vi "SendToBL_WeldAuto_Recipe.vi"(0 "connection ID":refnum<k5>, 1 "SC parameter to BL":string, 2 "MessageID_SC":i32, 7 "MessageID_PC_AC":i32, 9 "ResponseID":u8=66, 11 "Error IN":errorcluster, 12 "PC_AC parameter to BL":string) -> (4 "connection ID":refnum<k5>, 6 "Test status":string=" Success", 8 "String value response":string, 10 "Error OUT":errorcluster, 14 "SC Parameter written":i32, 15 "PC_AC parameter written":i32)   [LabVIEW 2017]
panel:
  out "*(type *) &x 2":u8
  out "*(type *) &x":u8
  # "INPUT"
  # "OUTPUT"
  # "Just for reference. Hence disabled"
  # "Read Me:\nThis VI will send the set of recipe parameters to \nSC BL and verifies the response recieved from the SCBL"
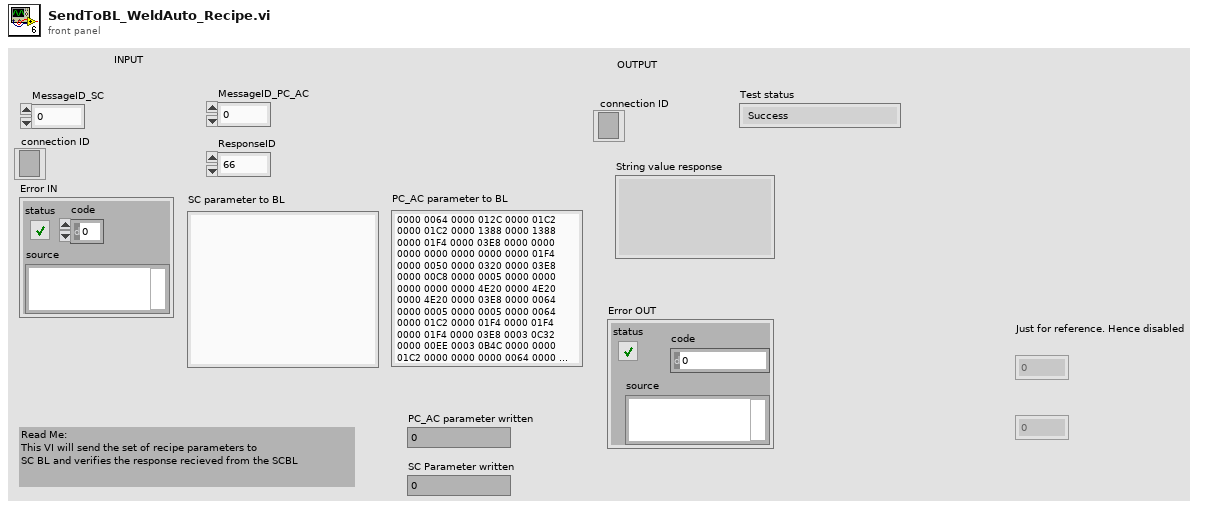
[diagram p1: front panel]
types:
  T1 = enum16{"big-endian, network order", "native, host order", "little-endian"}
  T2 = cluster{"SC parameter to BL":string, i32, "MessageID_SC":i32}
  T3 = cluster{"PC_AC parameter to BL":string, i32, "MessageID_PC_AC":i32}
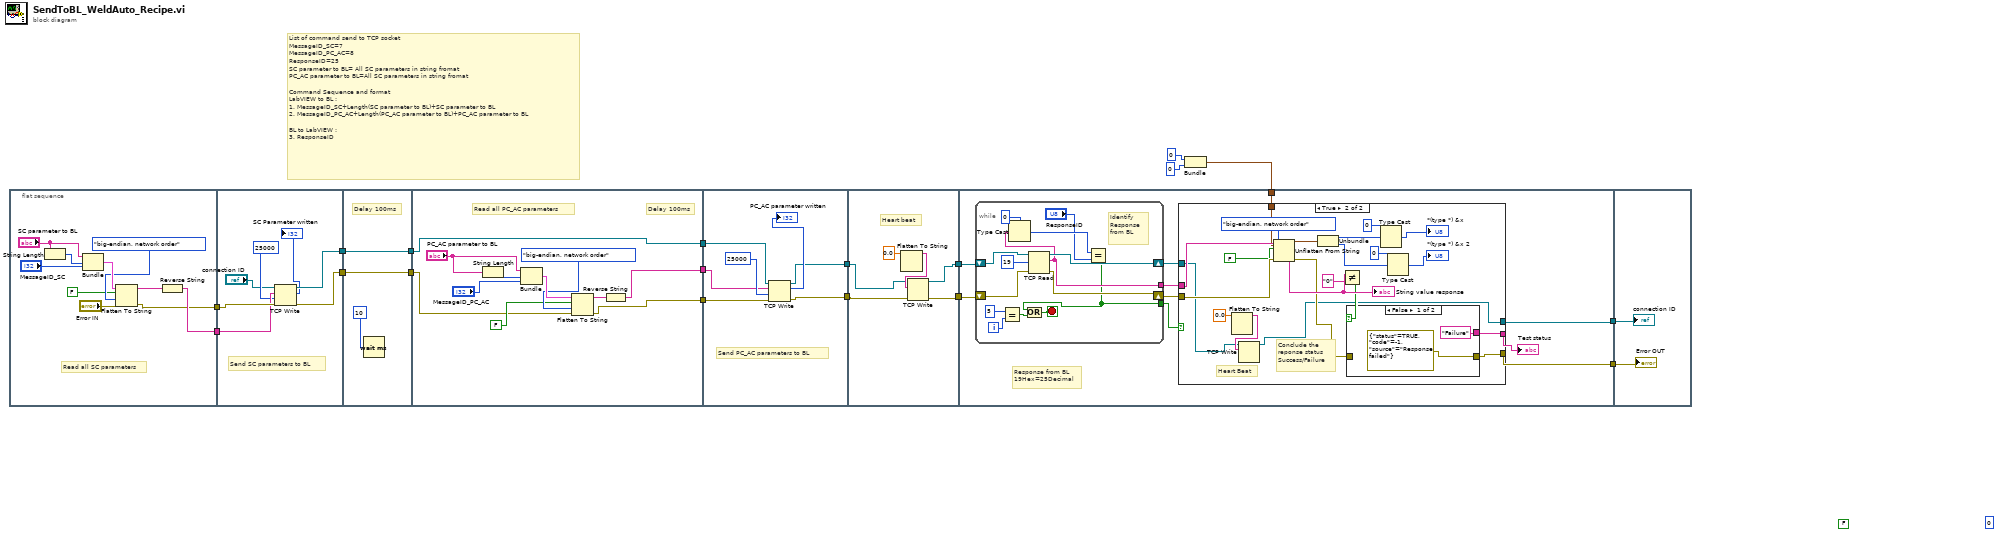
[diagram p0: block diagram]
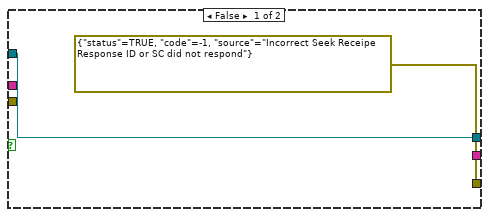
[diagram p2: hidden frame]
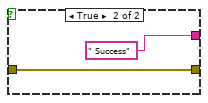
[diagram p3: hidden frame]
diagram:
  (unwired) u8 0
  (unwired) FALSE ("data includes array or string size? (T)")
  # "List of command send to TCP socket\nMessageID_SC=7\nMessageID_PC_AC=8\nResponseID=25\nSC parameter to BL= All SC parameters in string fromat\nPC_AC parameter to BL=All SC parameters in string fromat\n\nCommand Sequence and format\nLabVIEW to BL :\n1. MessageID_SC+Length(SC parameter to BL)+SC parameter to BL\n2. MessageID_PC_AC+Length(PC_AC parameter to BL)+PC_AC parameter to BL\n\nBL to LabVIEW :\n3. ResponseID"
  n1 = flat-sequence {
    tunnel: [w21] -> w11
    tunnel: [w22] -> w10
    tunnel: [w35] -> w18
    tunnel: [w34] -> w17
    tunnel: w11 -> [w33]
    tunnel: w10 -> [w32]
    tunnel: w18 -> [w38]
    tunnel: w17 -> [w37]
    tunnel: [w38] -> w9
    tunnel: [w37] -> w8
    tunnel: [w49] -> w7
    tunnel: [w48] -> w6
    tunnel: [w47] -> w5
    tunnel: w8 -> [w39]
    tunnel: w9 -> [w49]
    tunnel: [w51] -> w4
    tunnel: [w50] -> w2
    tunnel: w7 -> [w54]
    tunnel: w6 -> [w53]
    tunnel: w5 -> [w52]
    tunnel: w4 -> [w60]
    tunnel: [w58] -> w3
    tunnel: w2 -> [w59]
    tunnel: [w57] -> w1
    tunnel: w3 -> [w72]
    tunnel: w1 -> [w71]
    tunnel: w14 -> [w66]
    tunnel: [w65] -> w13
    tunnel: [w64] -> w12
    tunnel: w13 -> [w116]
    tunnel: w12 -> [w115]
    frame #0 {
      # "Read all SC parameters"
      n2 = String Length(string="SC parameter to BL") -> (length=w20:i32)
      n3 = Bundle("SC parameter to BL"="SC parameter to BL", w20, "MessageID_SC"="MessageID_SC") -> (w28:T2)  [unwired: 1 in]
      n4 = Flatten To String(anything=w28, prepend array or string size? (T)=FALSE, byte order (0:big-endian, network order)=T1."big-endian, network order", error in (no error)="Error IN") -> (data string=w25:string, error out=w21:errorcluster)  [unwired: 1 out]
      n5 = Reverse String(1:w25) -> (0:w22:string)
    }
    frame #1 {
      # "Send SC parameters to BL"
      n6 = TCP Write(connection ID="connection ID", data in=w32, error in (no error)=w33, 9:25000 ("timeout ms (25000)")) -> (connection ID out=w35:refnum<k5>, bytes written=→"SC Parameter written":i32, error out=w34:errorcluster)
    }
    frame #2 {
      # "Delay 100ms"
      n7 = Wait (ms)(milliseconds to wait=u32 10) -> ()  [unwired: 1 out]
    }
    frame #3 {
      # "Read all PC_AC parameters"
      # "Delay 100ms"
      n8 = String Length(string="PC_AC parameter to BL") -> (length=w41:i32)
      n9 = Bundle("PC_AC parameter to BL"="PC_AC parameter to BL", w41, "MessageID_PC_AC"="MessageID_PC_AC") -> (w46:T3)  [unwired: 1 in]
      n10 = Flatten To String(anything=w46, prepend array or string size? (T)=FALSE, byte order (0:big-endian, network order)=T1."big-endian, network order", error in (no error)=w39) -> (data string=w44:string, error out=w48:errorcluster)  [unwired: 1 out]
      n11 = Reverse String(1:w44) -> (0:w47:string)
    }
    frame #4 {
      # "Send PC_AC parameters to BL"
      n12 = TCP Write(connection ID=w54, data in=w52, error in (no error)=w53, 9:25000 ("timeout ms (25000)")) -> (connection ID out=w51:refnum<k5>, bytes written=→"PC_AC parameter written":i32, error out=w50:errorcluster)
    }
    frame #5 {
      # "Heart beat"
      n13 = Flatten To String(anything=0.0) -> (data string=w61:string)  [unwired: 3 in, 2 out]
      n14 = TCP Write(connection ID=w60, data in=w61, error in (no error)=w59) -> (connection ID out=w58:refnum<k5>, error out=w57:errorcluster)  [unwired: 1 in, 1 out]
    }
    frame #6 {
      # "Response from BL\n19Hex=25Decimal"
      n15 = while {
        tunnel: [w110] -> w69
        shift-right: [w112] -> w68
        shift-left: w72 -> [w114]
        shift-right: [w106] -> w70
        shift-left: w71 -> [w113]
        tunnel: [w104] -> w67
        i -> [w103]
        stop <- w105 stop-if-true
        # "Identify\nResponse \nfrom BL"
        n16 = Equal?(x=5, y=w103) -> (x = y?=w101:bool)
        n17 = TCP Read(connection ID=w114, bytes to read=19, error in (no error)=w113) -> (connection ID out=w112:refnum<k5>, data out=w110:string, error out=w106:errorcluster)  [unwired: 2 in]
        n18 = Type Cast(type=u8 0, x=w110) -> (*(type *) &x=w108:u8)
        n19 = Equal?(x=w108, y="ResponseID") -> (x = y?=w104:bool)
        n20 = Or(x=w104, y=w101) -> (x .or. y?=w105:bool)
      }
      n21 = case shown="True" w67 {
        tunnel: w70 -> [_ w96]
        tunnel: w69 -> [_ w95]
        tunnel: w68 -> [w74 w76]
        tunnel: w66 -> [_ w91]
        tunnel: [w74 w75] -> w65
        tunnel: [errorcluster {"status"=TRUE, "code"=-1, "source"="Incorrect Seek Receipe Response ID or SC did not respond"} ("error constant") w87] -> w64
        tunnel: [_ w86] -> w63
        frame False {
        }
        frame True {
          # "Heart Beat"
          # "Conclude the \nreponse status\nSuccess/Failure"
          n22 = Flatten To String(anything=0.0) -> (data string=w77:string)  [unwired: 3 in, 2 out]
          n23 = TCP Write(connection ID=w76, data in=w77) -> (connection ID out=w75:refnum<k5>)  [unwired: 2 in, 2 out]
          n24 = Unflatten From String(type=w91, binary string=w95, data includes array or string size? (T)=FALSE, byte order (0:big-endian, network order)=T1."big-endian, network order", error in (no error)=w96) -> (rest of the binary string=w90:string, value=w92:cluster{i32, i32}, error out=w85:errorcluster)
          "String value response" <- w90
          n25 = Unbundle(w92) -> (w84:i32, w79:i32)
          n26 = Not Equal?(x=w90, y="0") -> (x != y?=w88:bool)
          n27 = case shown="False" w88 {
            tunnel: [errorcluster {"status"=TRUE, "code"=-1, "source"="Response failed"} ("error constant") w99] -> w87
            tunnel: ["Failure" " Success"] -> w86
            tunnel: w85 -> [_ w99]
            frame False {
            }
            frame True {
            }
          }
          n28 = Type Cast(type=u8 0, x=w84) -> (*(type *) &x=→"*(type *) &x":u8)
          n29 = Type Cast(type=u8 0, x=w79) -> (*(type *) &x=→"*(type *) &x 2":u8)
        }
      }
      "Test status" <- w63
    }
    frame #7 {
      "connection ID" <- w116
      "Error OUT" <- w115
    }
  }
  n30 = Bundle(0, 0) -> (w14:cluster{i32, i32})  [unwired: 1 in]
